vi "BRig_Host_dataRunState__entryAdd__dataPlot_IdxColRow_get.vi"(5 "input_idx":i32[](array[numeric]), 7 "input_dataPlot":u16[][](array[numeric]), 10 "input_tSelectionPlot":u16, 11 "input_sSelection":u16) -> (1 "output_col_dataPlot":i32, 2 "output_row_dataPlot":i32, 3 "output_idx_dataPlot":i32)   [LabVIEW 2014]
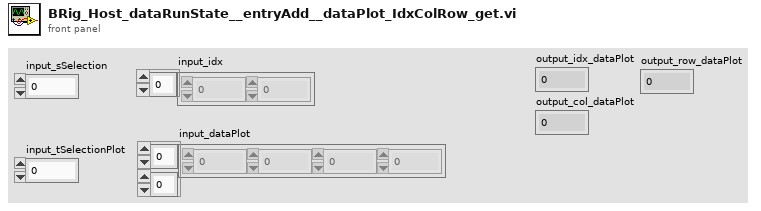
[diagram p1: front panel]
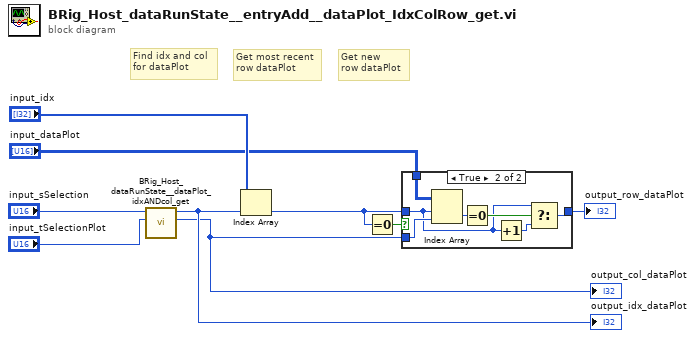
[diagram p0: block diagram]
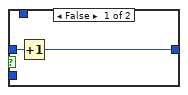
[diagram p2: hidden frame]
diagram:
  # "Get new\nrow dataPlot"
  # "Get most recent\nrow dataPlot"
  # "Find idx and col\nfor dataPlot"
  n1 = call "BRig_Host_dataRunState__dataPlot_idxANDcol_get.vi"("input_tSelection_plot"="input_tSelectionPlot", "input_sSelection"="input_sSelection") -> ("output_col_dataPlot"=w3:i32, "output_idx_dataPlot"=w6:i32)  [unwired: 8 in]
  "output_idx_dataPlot" <- w6
  "output_col_dataPlot" <- w3
  n2 = Index Array(array="input_idx", index=w6) -> (element=w4:i32)
  n3 = Equal To 0?(x=w4) -> (x = 0?=w5:bool)
  n4 = case shown="True" w5 {
    tunnel: "input_dataPlot" -> [_ w18]
    tunnel: w4 -> [w11 w12]
    tunnel: [w10 w13] -> w1
    tunnel: w3 -> [_ w17]
    frame False {
      n5 = Increment(x=w11) -> (x+1=w10:i32)
    }
    frame True {
      n6 = Index Array(array=w18, index (row)=w12, index (col)=w17) -> (element=w16:u16)
      n7 = Equal To 0?(x=w16) -> (x = 0?=w15:bool)
      n8 = Increment(x=w12) -> (x+1=w14:i32)
      n9 = Select(t=w12, s=w15, f=w14) -> (s? t:f=w13:i32)
    }
  }
  "output_row_dataPlot" <- w1
